vi "Stop Core.vi"(10 "final error code":i32, 11 "Task Setting Editor in":refnum<class "Task Setting Editor.lvclass">) -> (3 "Task Setting Editor out":refnum<class "Task Setting Editor.lvclass">)   [LabVIEW 2017, in "Task Setting Editor.lvlib" / "Task Setting Editor.lvclass"]
doc: "(<B>Filename</B>: Actor Framework.lvlib:Actor.lvclass:Stop Core.vi)\n\nDefines what the actor does before it stops. Use the <B>final error code</B> input to determine whether the actor shut down in response to an error.\n\nBy default, this method does nothing. A descendant class may override it to define behavior, such as shutting down any processes the actor initiated in its override of the Actor Core method."
uses:
  Task Setting Editor.lvclass
  Task Setting Editor.lvclass/Task Setting Editor.ctl
  Framework/Actor wHelper/Actor wHelper.lvclass
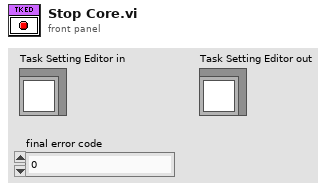
[diagram p1: front panel]
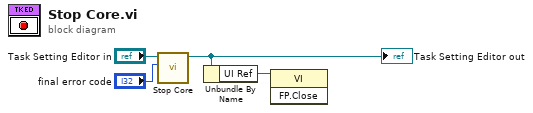
[diagram p0: block diagram]
diagram:
  n1 = call-parent "Stop Core.vi"("final error code"="final error code", "Actor wHelper in"="Task Setting Editor in") -> ("Actor wHelper out"=w2:refnum<class "Task Setting Editor.lvclass">)  [unwired: 9 in]
  "Task Setting Editor out" <- w2
  n2 = Unbundle By Name(w2) -> ("UI Ref"=w1:refnum<vi>)
  n3 = invoke class="VI" method="FP.Close"(reference=w1) -> ()  [unwired: 2 in, 3 out]
